vi "Debug_Convert_Data_to_String.vi"(8 "error in (no error)":errorcluster, 11 "AB_DLL in":refnum<class "AB_DLL.lvclass">) -> (0 "error out":errorcluster, 2 "classData":string, 3 "AB_DLL out":refnum<class "AB_DLL.lvclass">)   [LabVIEW 2020, in "AB_DLL.lvclass"]
uses:
  <vilib>/AppBuilder/AB_Classes/DLL/AB_DLL.lvclass
  <vilib>/AppBuilder/AB_Classes/DLL/AB_DLL.lvclass/AB_DLL.ctl
  <vilib>/AppBuilder/AB_Classes/Application/AB_Application.lvclass
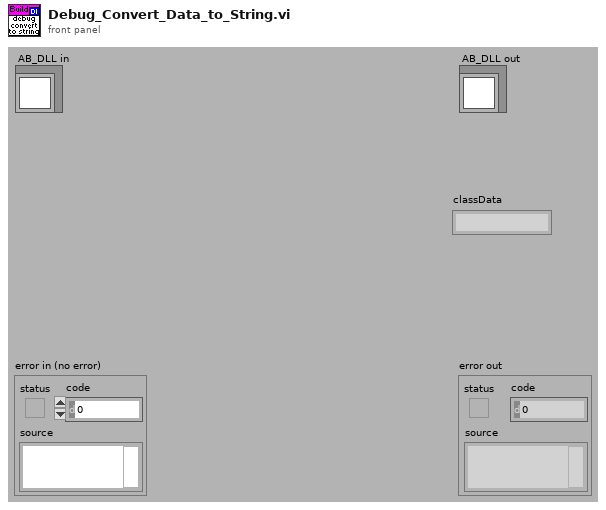
[diagram p1: front panel]
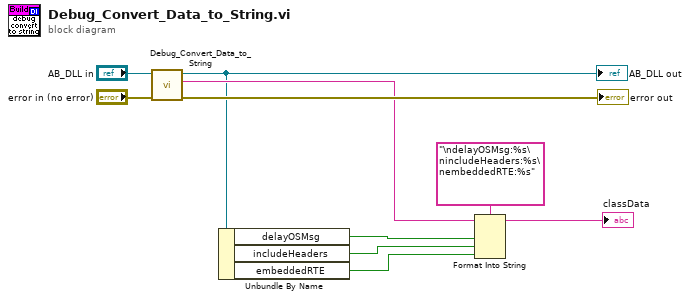
[diagram p0: block diagram]
diagram:
  n1 = call-parent "Debug_Convert_Data_to_String.vi"("error in (no error)"="error in (no error)", "AB_Application in"="AB_DLL in") -> ("error out"=→"error out":errorcluster, "classData"=w6:string, "AB_Application out"=w4:refnum<class "AB_DLL.lvclass">)  [unwired: 7 in]
  "AB_DLL out" <- w4
  n2 = Unbundle By Name(w4) -> ("delayOSMsg"=w3:bool, "includeHeaders"=w2:bool, "embeddedRTE"=w1:bool)
  n3 = Format Into String(format string="\ndelayOSMsg:%s\nincludeHeaders:%s\nembeddedRTE:%s", initial string=w6, w3, w2, w1) -> (resulting string=→"classData":string)  [unwired: 1 in, 1 out]
